vi "DS345 tw sonication.vi"(5 "Lasting time (s)":dbl=10.0, 7 "Apply force":bool, 8 "Cluster":T1={"Osc. Amp. (V)"=0.06, "Osc. Freq. (Hz)"=1200.0} {"Osc. Freq. (Hz)" min=1000.0 max=25000000.0 step=0.001 format="%.3f"; "Osc. Amp. (V)" min=0.01 max=10.0 step=0.01 format="%.3f"}, 9 "Default setting (DS345)":T1={"Osc. Amp. (V)"=0.01, "Osc. Freq. (Hz)"=1000.0} {"Osc. Freq. (Hz)" min=0.001 max=250000.0 step=0.001 format="%.3f"; "Osc. Amp. (V)" min=0.0 max=0.1 step=0.001 format="%.3f"}, 10 "SRS DS345 GPIB address":string="0:18") -> (0 "Status (s)":dbl)   [LabVIEW 2015]
panel:
  in  "stop":bool
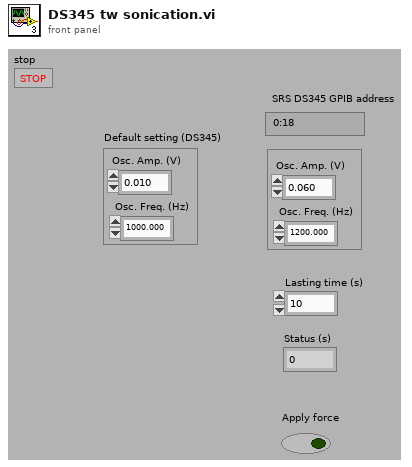
[diagram p1: front panel]
types:
  T1 = cluster{"Osc. Amp. (V)":dbl, "Osc. Freq. (Hz)":dbl}
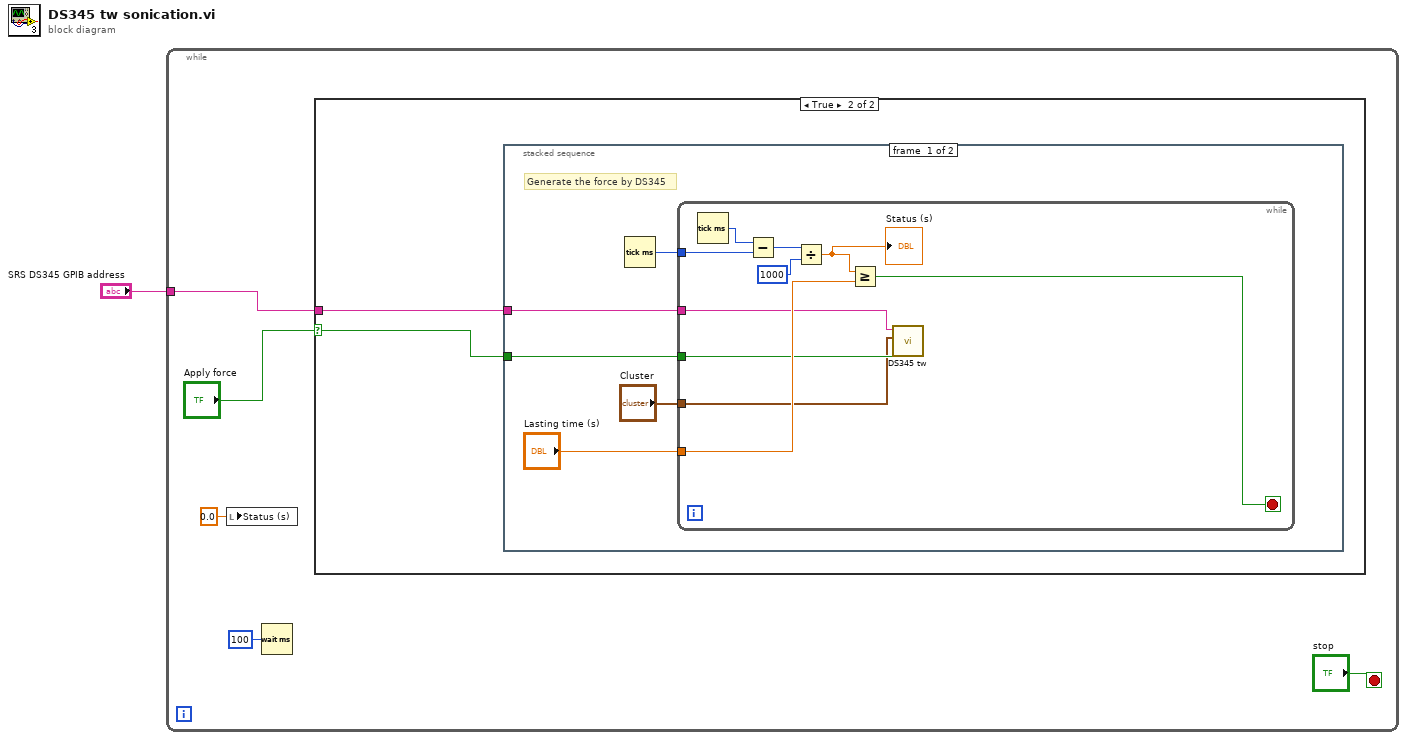
[diagram p0: block diagram]
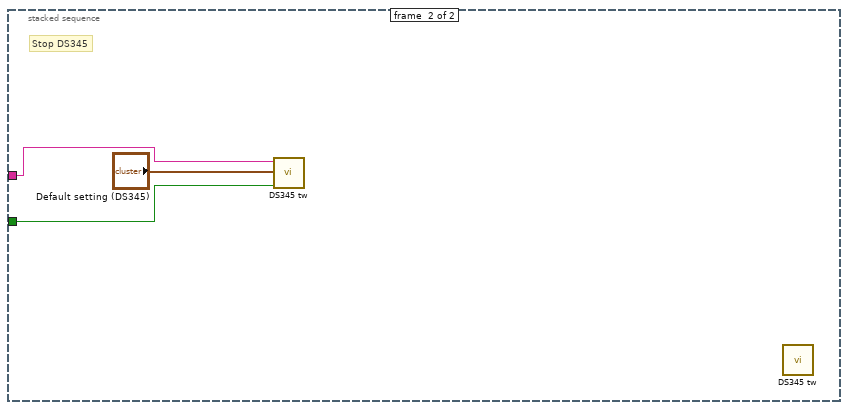
[diagram p3: hidden frame]
diagram:
  n1 = while {
    tunnel: "SRS DS345 GPIB address" -> [w6]
    stop <- "stop" stop-if-true
    n2 = local write "Status (s)"(0.0 ("Status (s)")) -> ()
    n3 = Wait (ms)(milliseconds to wait=u32 100) -> ()  [unwired: 1 out]
    n4 = case shown="True" "Apply force" {
      selector: "Apply force" -> [_ w8]
      tunnel: w6 -> [_ w7]
      frame False {
      }
      frame True {
        n5 = stacked-sequence {
          tunnel: w8 -> [w10 w24]
          tunnel: w7 -> [w11 w25]
          frame #0 {
            # "Generate the force by DS345"
            n6 = Tick Count (ms)() -> (millisecond timer value=w13:u32)
            n7 = while {
              tunnel: w13 -> [w22]
              tunnel: "Lasting time (s)" -> [w18]
              tunnel: w11 -> [w16]
              tunnel: w10 -> [w15]
              tunnel: "Cluster" -> [w14]
              stop <- w21 stop-if-true
              n8 = Tick Count (ms)() -> (millisecond timer value=w23:u32)
              n9 = Subtract(x=w23, y=w22) -> (x-y=w20:u32)
              n10 = Divide(x=w20, y=u32 1000) -> (x/y=w17:dbl)
              "Status (s)" <- w17
              n11 = Greater Or Equal?(x=w17, y=w18) -> (x >= y?=w21:bool)
              n12 = call "DS345 tw.vi"("Update"=w15, "Cluster"=w14, "SRS DS345 GPIB address"=w16) -> ()  [unwired: 9 in]
            }
          }
          frame #1 {
            # "Stop DS345"
            n13 = call "DS345 tw.vi"("Update"=w24, "Cluster"="Default setting (DS345)", "SRS DS345 GPIB address"=w25) -> ()  [unwired: 9 in]
            n14 = call "DS345 tw.vi"() -> ()  [unwired: 12 in]
          }
        }
      }
    }
  }
